vi "TRAFFIC LIGHT SUBVI.vi"() -> ()   [LabVIEW 2018]
panel:
  in  "Enum":enum16{"RED", "YELLOW", "GREEN"}(ring)
  out "GREEN":bool
  out "YELLOW":bool
  out "RED":bool
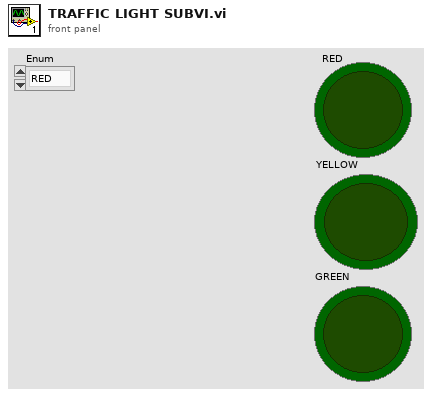
[diagram p1: front panel]
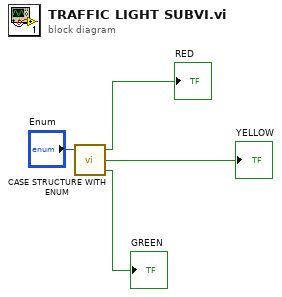
[diagram p0: block diagram]
diagram:
  n1 = call "CASE STRUCTURE WITH ENUM.vi"("Enum"="Enum") -> ("GREEN"=→"GREEN":bool, "YELLOW"=→"YELLOW":bool, "RED"=→"RED":bool)  [unwired: 2 in]
